vi "New.vi"(8 "error in (no error)":errorcluster, 10 "Topic":string, 11 "Subscription ID":u64) -> (0 "error out":errorcluster, 3 "SubscriptionDetails JSON out":refnum<class "SubscriptionDetails JSON.lvclass">)   [LabVIEW 2020, in "wamplv.lvlib" / "SubscriptionDetails JSON.lvclass"]
uses:
  SubscriptionDetails JSON.lvclass
  SubscriptionDetails JSON.lvclass/SubscriptionDetails JSON.ctl
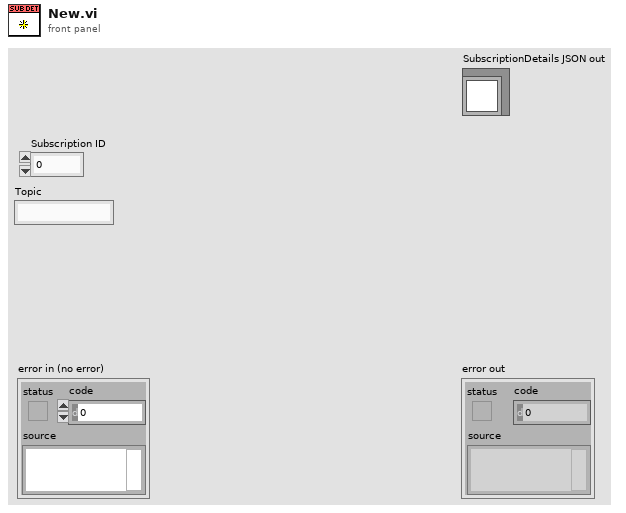
[diagram p1: front panel]
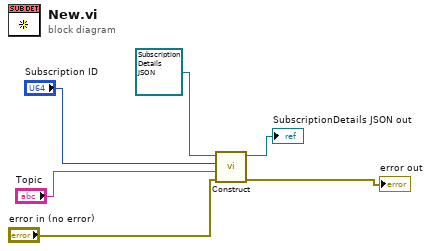
[diagram p0: block diagram]
diagram:
  n1 = call-dynamic "Construct.vi"("error in (no error)"="error in (no error)", "Topic"="Topic", "Subscription ID"="Subscription ID", "SubscriptionDetails JSON in"=refnum<class "SubscriptionDetails JSON.lvclass"> refnum) -> ("error out"=→"error out":errorcluster, "SubscriptionDetails JSON out"=→"SubscriptionDetails JSON out":refnum<class "SubscriptionDetails JSON.lvclass">)  [unwired: 6 in]
